vi "Percobaan 1.vi"() -> ()   [LabVIEW 2020]
uses:
  <vilib>/MakerHub/LINX/Public/Peripherals/Analog/Analog Read 1 Chan.vi
  <vilib>/MakerHub/LINX/Public/Peripherals/Digital/Digital Write 1 Chan.vi
  <vilib>/MakerHub/LINX/Public/Peripherals/Analog/Analog Read N Chans.vi
  <vilib>/MakerHub/LINX/Public/Peripherals/Digital/Digital Write N Chans.vi
  <vilib>/MakerHub/LINX/Private/Local IO/LinxAnalogRead.vi
  <vilib>/MakerHub/LINX/Public/Utilities/Check Channel.vi
  <vilib>/MakerHub/LINX/Private/Local IO/LinxDigitalWrite.vi
  <vilib>/MakerHub/LINX/Public/Utilities/Open Serial.vi
  <vilib>/MakerHub/LINX/Private/Utilties/Generate Error.vi
  <vilib>/MakerHub/LINX/LMH-LINX.lvlib
panel:
  out "Waveform Chart 2":dbl(graph)
  out "ON/OFF":bool
  out "suhu":dbl(knob) scale=0.0..100.0
  in  "stop":bool
  in  "Serial Port":refnum<visa-resource-name>
  # "MONITORING SENSOR SUHU LM PADA LABVIEW"
  # "EK-2B\n1. Aldisyah Putra Mahardika   \t\t\n(EK-2B/3.32.21.1.02) \n2. Aurelia Alika Putri Widiyanta  \t\n(EK-2B/3.32.21.1.04) \n3. Fahmi Fathur Rohman     \t\t\n(EK-2B/3.32.21.1.08)"
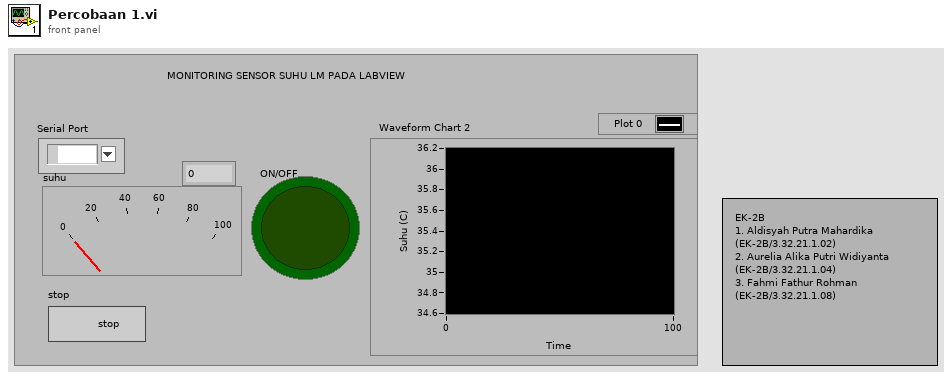
[diagram p1: front panel]
types:
  T1 = typedef "LMH-LINX.lvlib/LINX Ref.ctl" = cluster{"IO":T2, "Interface":T3, "LINX Device Config":T4}
  T2 = typedef "LMH-LINX.lvlib/Platform.ctl" = enum16{"Remote", "Local"}
  T3 = typedef "LMH-LINX.lvlib/Interface.ctl" = enum16{"Serial", "TCP"}
  T4 = typedef "LMH-LINX.lvlib/Device.lvlib/LINX Device Config.ctl" = cluster{"Interface":T3, "COM Port":refnum<visa-resource-name>, "TCP Configuration":T5, "Device Family":u8, "Device ID":u8, "Device Name":string, "TCP Ref":refnum<k5>, "Channels":T6}
  T5 = typedef "LMH-LINX.lvlib/Device.lvlib/TCP Config.ctl" = cluster{"IP Address":string, "Port":u16}
  T6 = typedef "LMH-LINX.lvlib/Channels.ctl" = cluster{"DI":u8[], "DO":u8[], "AI":u8[], "AO":u8[], "PWM":u8[], "QE":u8[], "UART":u8[], "I2C 2":u8[], "SPI":u8[], "CAN":u8[], "Servo":u8[], "AI Ref (V)":dbl, "AI Resolution (Bits)":u8, "AO Ref (V)":dbl, "AO Resolution (Bits)":u8}
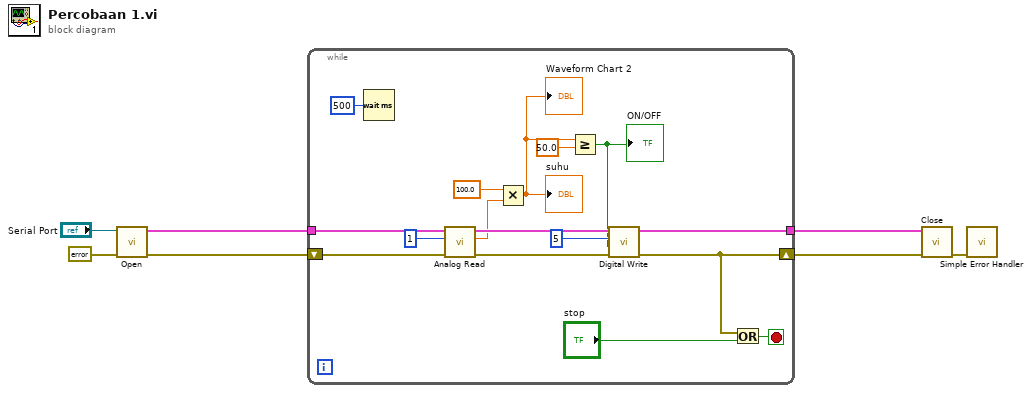
[diagram p0: block diagram]
diagram:
  n1 = call-poly <vilib>:"Open.vi"("Error In"=errorcluster {"status"=FALSE, "code"=0, "source"=""}, "Serial Port"="Serial Port") -> ("Error Out"=w6:errorcluster, "LINX Resource"=w7:T1)  [unwired: 7 in, 1 out]
  n2 = while {
    tunnel: w7 -> [w22]
    shift-right: [w17] -> w5
    shift-left: w6 -> [w21]
    tunnel: [w18] -> w1
    stop <- w23 stop-if-true
    n3 = Wait (ms)(milliseconds to wait=u32 500) -> ()  [unwired: 1 out]
    n4 = call-poly <vilib>:"Analog Read.vi"("Error In"=w21, "Analog Channel"=u8 1, "LINX Resource"=w22) -> ("Error Out"=w16:errorcluster, "Voltage"=w9:dbl, "LINX Resource"=w14:T1)  [unwired: 5 in, 1 out]
    n5 = Multiply(x=100.0, y=w9) -> (x*y=w8:dbl)
    "suhu" <- w8
    "Waveform Chart 2" <- w8
    n6 = Greater Or Equal?(x=w8, y=50.0) -> (x >= y?=w12:bool)
    "ON/OFF" <- w12
    n7 = call-poly <vilib>:"Digital Write.vi"("Error In"=w16, "Output Value"=w12, "DO Channel"=u8 5, "LINX Resource"=w14) -> ("Error Out"=w17:errorcluster, "LINX Resource"=w18:T1)  [unwired: 6 in]
    n8 = Or(x=w17, y="stop") -> (x .or. y?=w23:bool)
  }
  n9 = call <vilib>:"Close.vi"("Error In"=w5, "LINX Resource"=w1) -> ("Error Out"=w3:errorcluster)  [unwired: 9 in]
  n10 = call <vilib>:"Simple Error Handler.vi"("error in (no error)"=w3) -> ()  [unwired: 4 in, 5 out]
